vi "barcode inc.vi"() -> ()   [LabVIEW 2015]
panel:
  out "go in printer":string="0166"
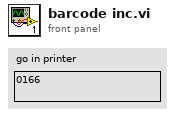
[diagram p1: front panel]
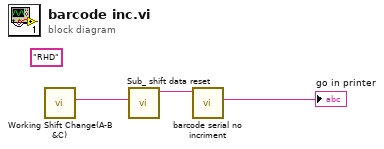
[diagram p0: block diagram]
diagram:
  (unwired) "RHD" ("Model Name")
  n1 = call "Working Shift Change(A-B &C).vi"() -> ("Shift Change"=w3:string)  [unwired: 9 in]
  n2 = call "Sub_ shift data reset.vi"("Shift"=w3) -> ("Serial no"=w2:string)  [unwired: 8 in, 1 out]
  n3 = call "barcode serial no incriment.vi"("Serial No"=w2) -> ("go in printer"=→"go in printer":string)  [unwired: 9 in, 1 out]
